vi "Ballard - Arinc-429 - Clear Database.vi"(8 "error in (no error)":errorcluster, 11 "Node Ptr":u64 format="%.0x") -> (0 "error out":errorcluster)   [LabVIEW 2016, in "Ballard Arinc-429 System Explorer.lvlib"]
uses:
  Ballard Arinc-429 System Explorer.lvlib
  <vilib>/NI VeriStand/Custom Device API/Custom Device API.lvlib
  Shared/Controls and Global/Global.vi
  Shared/Ballard Arinc-429 Shared.lvlib
  <vilib>/NI VeriStand/Custom Device Tools/Custom Device Utility Library/Custom Device Utility Library.lvlib
  <vilib>/NI Veristand/Custom Device Tools/Custom Device Utility Library/NI VeriStand - Search for Item by GUID.vi
panel:
  in  "Tag":string
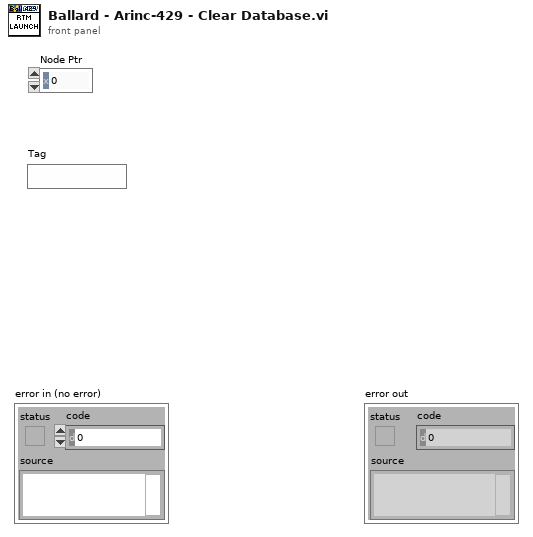
[diagram p1: front panel]
types:
  T1 = typedef "Custom Device API.lvlib/Custom Device Item Ref.ctl" = u64
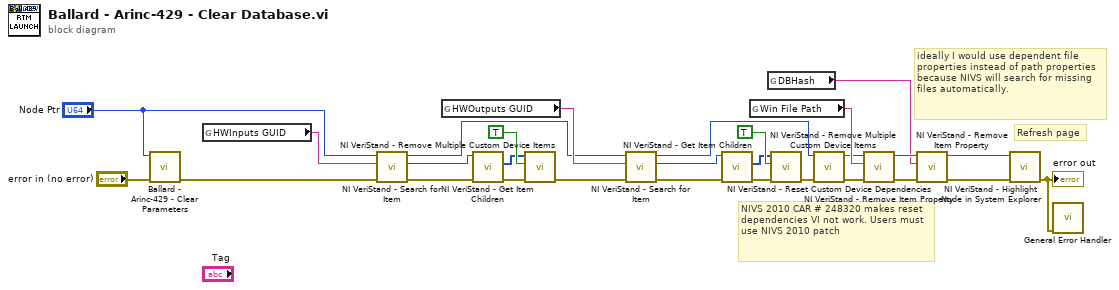
[diagram p0: block diagram]
diagram:
  # "ideally I would use dependent file properties instead of path properties because NIVS will search for missing files automatically."
  # "NIVS 2010 CAR # 248320 makes reset dependencies VI not work. Users must use NIVS 2010 patch"
  # "Refresh page"
  n1 = call "Ballard - Arinc-429 - Clear Parameters.vi"("error in (no error)"="error in (no error)", "Node Ptr"="Node Ptr") -> ("error out"=w2:errorcluster)  [unwired: 9 in]
  n2 = global read "Global.vi" "HWInputs GUID"() -> (w22:string)
  n3 = call-poly <vilib>:"NI VeriStand - Search for Item.vi"("error in"=w2, "Item GUID"=w22, "Section Ref in"="Node Ptr") -> ("error out"=w18:errorcluster, "Item Ref"=w21:T1, "Section Ref out"=w11:T1)  [unwired: 5 in, 1 out]
  n4 = global read "Global.vi" "HWOutputs GUID"() -> (w16:string)
  n5 = call <vilib>:"NI VeriStand - Get Item Children.vi"("error in (no error)"=w18, "Item Ref in"=w21) -> ("error out"=w28:errorcluster, "Child Refs"=w23:T1[])  [unwired: 6 in, 2 out]
  n6 = call <vilib>:"NI VeriStand - Remove Multiple Custom Device Items.vi"("error in (no error)"=w28, "Force Delete (F)"=TRUE, "Item Refs in"=w23) -> ("error out"=w17:errorcluster)  [unwired: 7 in, 1 out]
  n7 = call-poly <vilib>:"NI VeriStand - Search for Item.vi"("error in"=w17, "Item GUID"=w16, "Section Ref in"=w11) -> ("error out"=w14:errorcluster, "Item Ref"=w15:T1, "Section Ref out"=w10:T1)  [unwired: 5 in, 1 out]
  n8 = call <vilib>:"NI VeriStand - Get Item Children.vi"("error in (no error)"=w14, "Item Ref in"=w15) -> ("error out"=w19:errorcluster, "Child Refs"=w13:T1[])  [unwired: 6 in, 2 out]
  n9 = global read "Global.vi" "Win File Path"() -> (w25:string)
  n10 = global read "Global.vi" "DBHash"() -> (w4:string)
  n11 = call <vilib>:"NI VeriStand - Remove Multiple Custom Device Items.vi"("error in (no error)"=w19, "Force Delete (F)"=TRUE, "Item Refs in"=w13) -> ("error out"=w12:errorcluster)  [unwired: 7 in, 1 out]
  n12 = call <vilib>:"NI VeriStand - Reset Custom Device Dependencies.vi"("error in (no error)"=w12, "Device Ref in"=w10) -> ("error out"=w26:errorcluster, "Device Ref out"=w24:T1)  [unwired: 8 in]
  n13 = call <vilib>:"NI VeriStand - Remove Item Property.vi"("error in (no error)"=w26, "Property Name"=w25, "Item Ref in"=w24) -> ("error out"=w8:errorcluster, "Item Ref out"=w7:T1)  [unwired: 6 in, 1 out]
  n14 = call <vilib>:"NI VeriStand - Remove Item Property.vi"("error in (no error)"=w8, "Property Name"=w4, "Item Ref in"=w7) -> ("error out"=w6:errorcluster, "Item Ref out"=w5:T1)  [unwired: 6 in, 1 out]
  n15 = call <vilib>:"NI VeriStand - Highlight Node in System Explorer.vi"("error in (no error)"=w6, "Item Ref in"=w5) -> ("error out"=w9:errorcluster)  [unwired: 8 in, 1 out]
  "error out" <- w9
  n16 = call <vilib>:"General Error Handler.vi"("error in (no error)"=w9) -> ()  [unwired: 10 in, 5 out]
